vi "Load Program.vi"(7 "Queue in":refnum<queue>, 8 "error in (no error)":errorcluster, 9 "Program Filepath":path, 10 "HW Settings in":T7={"Bike Parameters"={"Bike Simulated?"=enum."Simulated", "COM Port"="", "Baud Rate"=0}, "Crank Motor Parameters"={"Crank Motor Simulated?"=enum."Simulated", "Crank Motor COM Port"="", "Unit ID"=0, "Baud Rate"=0, "Parity (Odd)"=enum."None", "Serial Type"=enum."RTU", "Flow Control (none)"=enum."None"}, "Resistance Parameters"={"Resistance Simulated?"=enum."Simulated", "Resistance COM Port"="", "Baud Rate"=0, "Flow Control (none)"=0, "Default Velocity (RPM)"=0.0, "Motor Address"=0, "Data Bits (8)"=0, "Parity (0:none)"=0, "Stop Bits"=0, "Resistance Motor Parameters"={"Command Mode"=0, "#Step/per Rev"=0, "Protocol Mode"=0, "Max Accel.(rev/sec/sec)"=0, "Jog Speed(rev/sec)"=0.0, "Decel Rate(rev/sec/sec)"=0, "Power Up Current(A)"=0.0, "Idle Current(A)"=0.0, "Position Fault(%)"=0, "Power Mode"=0, "Proportional Gain"=0.03, "Min Speed (rps)"=0.03, "Resistance Acceptance"=[]}, "Default Timeout (ms)"=0, "Log Resistance Motion"=FALSE}, "Acquisition Parameters"={"Acquisition Simulated?"=enum."Simulated", "Sample Rate"=0.0, "Torque AI Channel"="cDAQ1Mod1/ai0", "TC 1 Channel"="cDAQ1Mod2/ai0", "TC 2 Channel"="cDAQ1Mod2/ai0", "Torque CCW Polynomial Coeff (V to Nm)"=[], "Torque CW Polynomial Coeff (V to Nm)"=[], "Max Torque (Nm)"=0.0, "Min Torque (Nm)"=0.0, "B Input Terminal"="/cDAQ1Mod2/PFI1", "A Input Terminal"="/cDAQ1Mod2/PFI0", "Motor RPM Counter"="cDAQ1Mod2/ai0", "Motor Timing Counter"="cDAQ1Mod2/ctr0", "Motor Internal Output"="/cDAQ1/Ctr1InternalOutput", "Servo Encoder Pulses per Revolution"=2500, "Dyno Power Smoothing Time (s) for display only"=0.0, "Dyno Torque Tare Smoothing Time (s)"=2.0, "Power Error Smoothing Time (s) for display only"=0.0}, "Default Program Folder"=path "", "Program Filepath"=path "", "Program Changed?"=FALSE, "Plot Categories"=[]} {"Acquisition Parameters"."Power Error Smoothing Time (s) for display only" min=0.1; "Acquisition Parameters"."Dyno Power Smoothing Time (s) for display only" min=0.1; "Acquisition Parameters"."Torque CW Polynomial Coeff (V to Nm)" format="%.6e"; "Acquisition Parameters"."Torque CCW Polynomial Coeff (V to Nm)" format="%.6e"; "Resistance Parameters"."Stop Bits" items=["1.0"=10, "1.5"=15, "2.0"=20]; "Resistance Parameters"."Parity (0:none)" items=["None", "Odd", "Even", "Mark", "Space"]; "Resistance Parameters"."Data Bits (8)" min=5 max=8 step=1; "Resistance Parameters"."Flow Control (none)" items=["None", "XON/XOFF", "RTS/CTS", "XON/XOFF & RTS/CTS", "DTR/DSR", "XON/XOFF & DTR/DSR"]}, 11 "Program in":T1={"Raw Logging Configuration"={"Log File Base Path"=path ""}, "Sequence"={"Start RPM"=0.0, "End RPM"=0.0, "# RPM Steps"=0, "Dwell (s)"=0.0, "Start L-value / Resist"=0, "End L-value/Resist"=0, "# L-value/Resist Steps"=0, "Steady State +/-RPM"=0.0, "Enable Steady State +/- RPM"=FALSE, "Steady State Window (s)"=0.0, "Enable Steady State Max Wait"=FALSE, "Max Settle Time (s)"=0.0, "Enable Temperature Rest"=FALSE, "Rest TC2 threshold (degF)"=2.0, "Enable Max Time Rest"=FALSE, "Max Rest Time (s)"=10.0, "Rest RPM"=2.0, "RPM Ramp (rpm/s)"=10.0, "Resistance Motor Mode"=enum."v1 Bike"}, "Summary  CSV Log Configuration"={"Report  CSV File Path"=path "", "Enable Report CSV File"=FALSE}, "CSV Log Info"={"Report Title"="", "Time Stamp"=timestamp(0 s since 1904-01-01), "Serial Number"="", "Initial Temperature"=0.0, "Comments"=""}, "Table"=[]} {"Sequence"."RPM Ramp (rpm/s)" min=0.0 format="%#_6f"; "Sequence"."Rest RPM" min=0.0 format="%.1f"; "Sequence"."Max Rest Time (s)" min=0.0 format="%.1f"; "Sequence"."Rest TC2 threshold (degF)" format="%.1f"; "Sequence"."Max Settle Time (s)" min=0.0 format="%.1f"; "Sequence"."Steady State Window (s)" min=0.0 format="%.1f"; "Sequence"."Steady State +/-RPM" min=0.0 format="%.1f"; "Sequence"."# L-value/Resist Steps" min=1; "Sequence"."End L-value/Resist" min=0 max=100; "Sequence"."Start L-value / Resist" min=0 max=100; "Sequence"."Dwell (s)" min=0.0 format="%#_6f"; "Sequence"."# RPM Steps" min=1; "Sequence"."End RPM" min=0.0 max=200.0 format="%#_6f"; "Sequence"."Start RPM" min=0.0 max=200.0 format="%#_6f"}) -> (0 "error out":errorcluster, 2 "HW Settings out":T7={"Bike Parameters"={"Bike Simulated?"=enum."Simulated", "COM Port"="", "Baud Rate"=0}, "Crank Motor Parameters"={"Crank Motor Simulated?"=enum."Simulated", "Crank Motor COM Port"="", "Unit ID"=0, "Baud Rate"=0, "Parity (Odd)"=enum."None", "Serial Type"=enum."RTU", "Flow Control (none)"=enum."None"}, "Resistance Parameters"={"Resistance Simulated?"=enum."Simulated", "Resistance COM Port"="", "Baud Rate"=0, "Flow Control (none)"=0, "Default Velocity (RPM)"=0.0, "Motor Address"=0, "Data Bits (8)"=0, "Parity (0:none)"=0, "Stop Bits"=0, "Resistance Motor Parameters"={"Command Mode"=0, "#Step/per Rev"=0, "Protocol Mode"=0, "Max Accel.(rev/sec/sec)"=0, "Jog Speed(rev/sec)"=0.0, "Decel Rate(rev/sec/sec)"=0, "Power Up Current(A)"=0.0, "Idle Current(A)"=0.0, "Position Fault(%)"=0, "Power Mode"=0, "Proportional Gain"=0.03, "Min Speed (rps)"=0.03, "Resistance Acceptance"=[]}, "Default Timeout (ms)"=0, "Log Resistance Motion"=FALSE}, "Acquisition Parameters"={"Acquisition Simulated?"=enum."Simulated", "Sample Rate"=0.0, "Torque AI Channel"="cDAQ1Mod1/ai0", "TC 1 Channel"="cDAQ1Mod2/ai0", "TC 2 Channel"="cDAQ1Mod2/ai0", "Torque CCW Polynomial Coeff (V to Nm)"=[], "Torque CW Polynomial Coeff (V to Nm)"=[], "Max Torque (Nm)"=0.0, "Min Torque (Nm)"=0.0, "B Input Terminal"="/cDAQ1Mod2/PFI1", "A Input Terminal"="/cDAQ1Mod2/PFI0", "Motor RPM Counter"="cDAQ1Mod2/ai0", "Motor Timing Counter"="cDAQ1Mod2/ctr0", "Motor Internal Output"="/cDAQ1/Ctr1InternalOutput", "Servo Encoder Pulses per Revolution"=2500, "Dyno Power Smoothing Time (s) for display only"=0.0, "Dyno Torque Tare Smoothing Time (s)"=2.0, "Power Error Smoothing Time (s) for display only"=0.0}, "Default Program Folder"=path "", "Program Filepath"=path "", "Program Changed?"=FALSE, "Plot Categories"=[]} {"Acquisition Parameters"."Power Error Smoothing Time (s) for display only" min=0.1; "Acquisition Parameters"."Dyno Power Smoothing Time (s) for display only" min=0.1; "Acquisition Parameters"."Torque CW Polynomial Coeff (V to Nm)" format="%.6e"; "Acquisition Parameters"."Torque CCW Polynomial Coeff (V to Nm)" format="%.6e"; "Resistance Parameters"."Stop Bits" items=["1.0"=10, "1.5"=15, "2.0"=20]; "Resistance Parameters"."Parity (0:none)" items=["None", "Odd", "Even", "Mark", "Space"]; "Resistance Parameters"."Data Bits (8)" min=5 max=8 step=1; "Resistance Parameters"."Flow Control (none)" items=["None", "XON/XOFF", "RTS/CTS", "XON/XOFF & RTS/CTS", "DTR/DSR", "XON/XOFF & DTR/DSR"]}, 3 "Program out":T1={"Raw Logging Configuration"={"Log File Base Path"=path ""}, "Sequence"={"Start RPM"=0.0, "End RPM"=0.0, "# RPM Steps"=0, "Dwell (s)"=0.0, "Start L-value / Resist"=0, "End L-value/Resist"=0, "# L-value/Resist Steps"=0, "Steady State +/-RPM"=0.0, "Enable Steady State +/- RPM"=FALSE, "Steady State Window (s)"=0.0, "Enable Steady State Max Wait"=FALSE, "Max Settle Time (s)"=0.0, "Enable Temperature Rest"=FALSE, "Rest TC2 threshold (degF)"=2.0, "Enable Max Time Rest"=FALSE, "Max Rest Time (s)"=10.0, "Rest RPM"=2.0, "RPM Ramp (rpm/s)"=10.0, "Resistance Motor Mode"=enum."v1 Bike"}, "Summary  CSV Log Configuration"={"Report  CSV File Path"=path "", "Enable Report CSV File"=FALSE}, "CSV Log Info"={"Report Title"="", "Time Stamp"=timestamp(0 s since 1904-01-01), "Serial Number"="", "Initial Temperature"=0.0, "Comments"=""}, "Table"=[]} {"Sequence"."RPM Ramp (rpm/s)" min=0.0 format="%#_6f"; "Sequence"."Rest RPM" min=0.0 format="%.1f"; "Sequence"."Max Rest Time (s)" min=0.0 format="%.1f"; "Sequence"."Rest TC2 threshold (degF)" format="%.1f"; "Sequence"."Max Settle Time (s)" min=0.0 format="%.1f"; "Sequence"."Steady State Window (s)" min=0.0 format="%.1f"; "Sequence"."Steady State +/-RPM" min=0.0 format="%.1f"; "Sequence"."# L-value/Resist Steps" min=1; "Sequence"."End L-value/Resist" min=0 max=100; "Sequence"."Start L-value / Resist" min=0 max=100; "Sequence"."Dwell (s)" min=0.0 format="%#_6f"; "Sequence"."# RPM Steps" min=1; "Sequence"."End RPM" min=0.0 max=200.0 format="%#_6f"; "Sequence"."Start RPM" min=0.0 max=200.0 format="%#_6f"})   [LabVIEW 2021, in "Config Module.lvlib"]
uses:
  Config Module.lvlib
  Controls/Config File Operation Enum.ctl
  support/Message Queue/Enqueue Message (Single).vi
  support/Message Queue/Message Cluster.ctl
  Peloton Bike/Signal Type.ctl
  Peloton Bike/Bike Parameters.ctl
  Crank Motor/Signal Type.ctl
  Crank Motor/Crank Motor Parameters.ctl
  Resistance Motor/Signal Type.ctl
  Resistance Motor/Resistance Motor Default Params.ctl
  Resistance Motor/Resistance Parameters.ctl
  Acquisition/Signal Type.ctl
  Acquisition/Acquisition Parameters.ctl
  Settings/Settings.ctl
  Settings/Settings.lvlib
  Logging/Logging Configuration.ctl
  Logging/Logging.lvlib
  Settings/Sequence Cluster.ctl
  controls/CSV Log Cluster.ctl
  Settings/Program Cluster.ctl
  controls/CSV Log Info Cluster.ctl
  Graph Folder/History Graph/Controls/Plot Category Cluster.ctl
  Resistance Motor/Resistance Mode Enum.ctl
  Resistance Motor/Resistance Acceptance Range.ctl
panel:
  # "Settled when"
  # "RPM is within"
  # "RPM of set RPM for last"
  # "seconds"
  # "OR"
  # "seconds since last step change"
  # "More than"
  # "Rest at end of each step at"
  # "RPM until"
  # "TC2 temperature is below"
  # "deg F"
  # "OR"
  # "seconds have elapsed"
  # "More than"
  # "Settled when"
  # "RPM is within"
  # "RPM of set RPM for last"
  # "seconds"
  # "OR"
  # "seconds since last step change"
  # "More than"
  # "Rest at end of each step at"
  # "RPM until"
  # "TC2 temperature is below"
  # "deg F"
  # "OR"
  # "seconds have elapsed"
  # "More than"
  # "(Silicon Labs CP210x)"
  # "(Silicon Labs CP210x)"
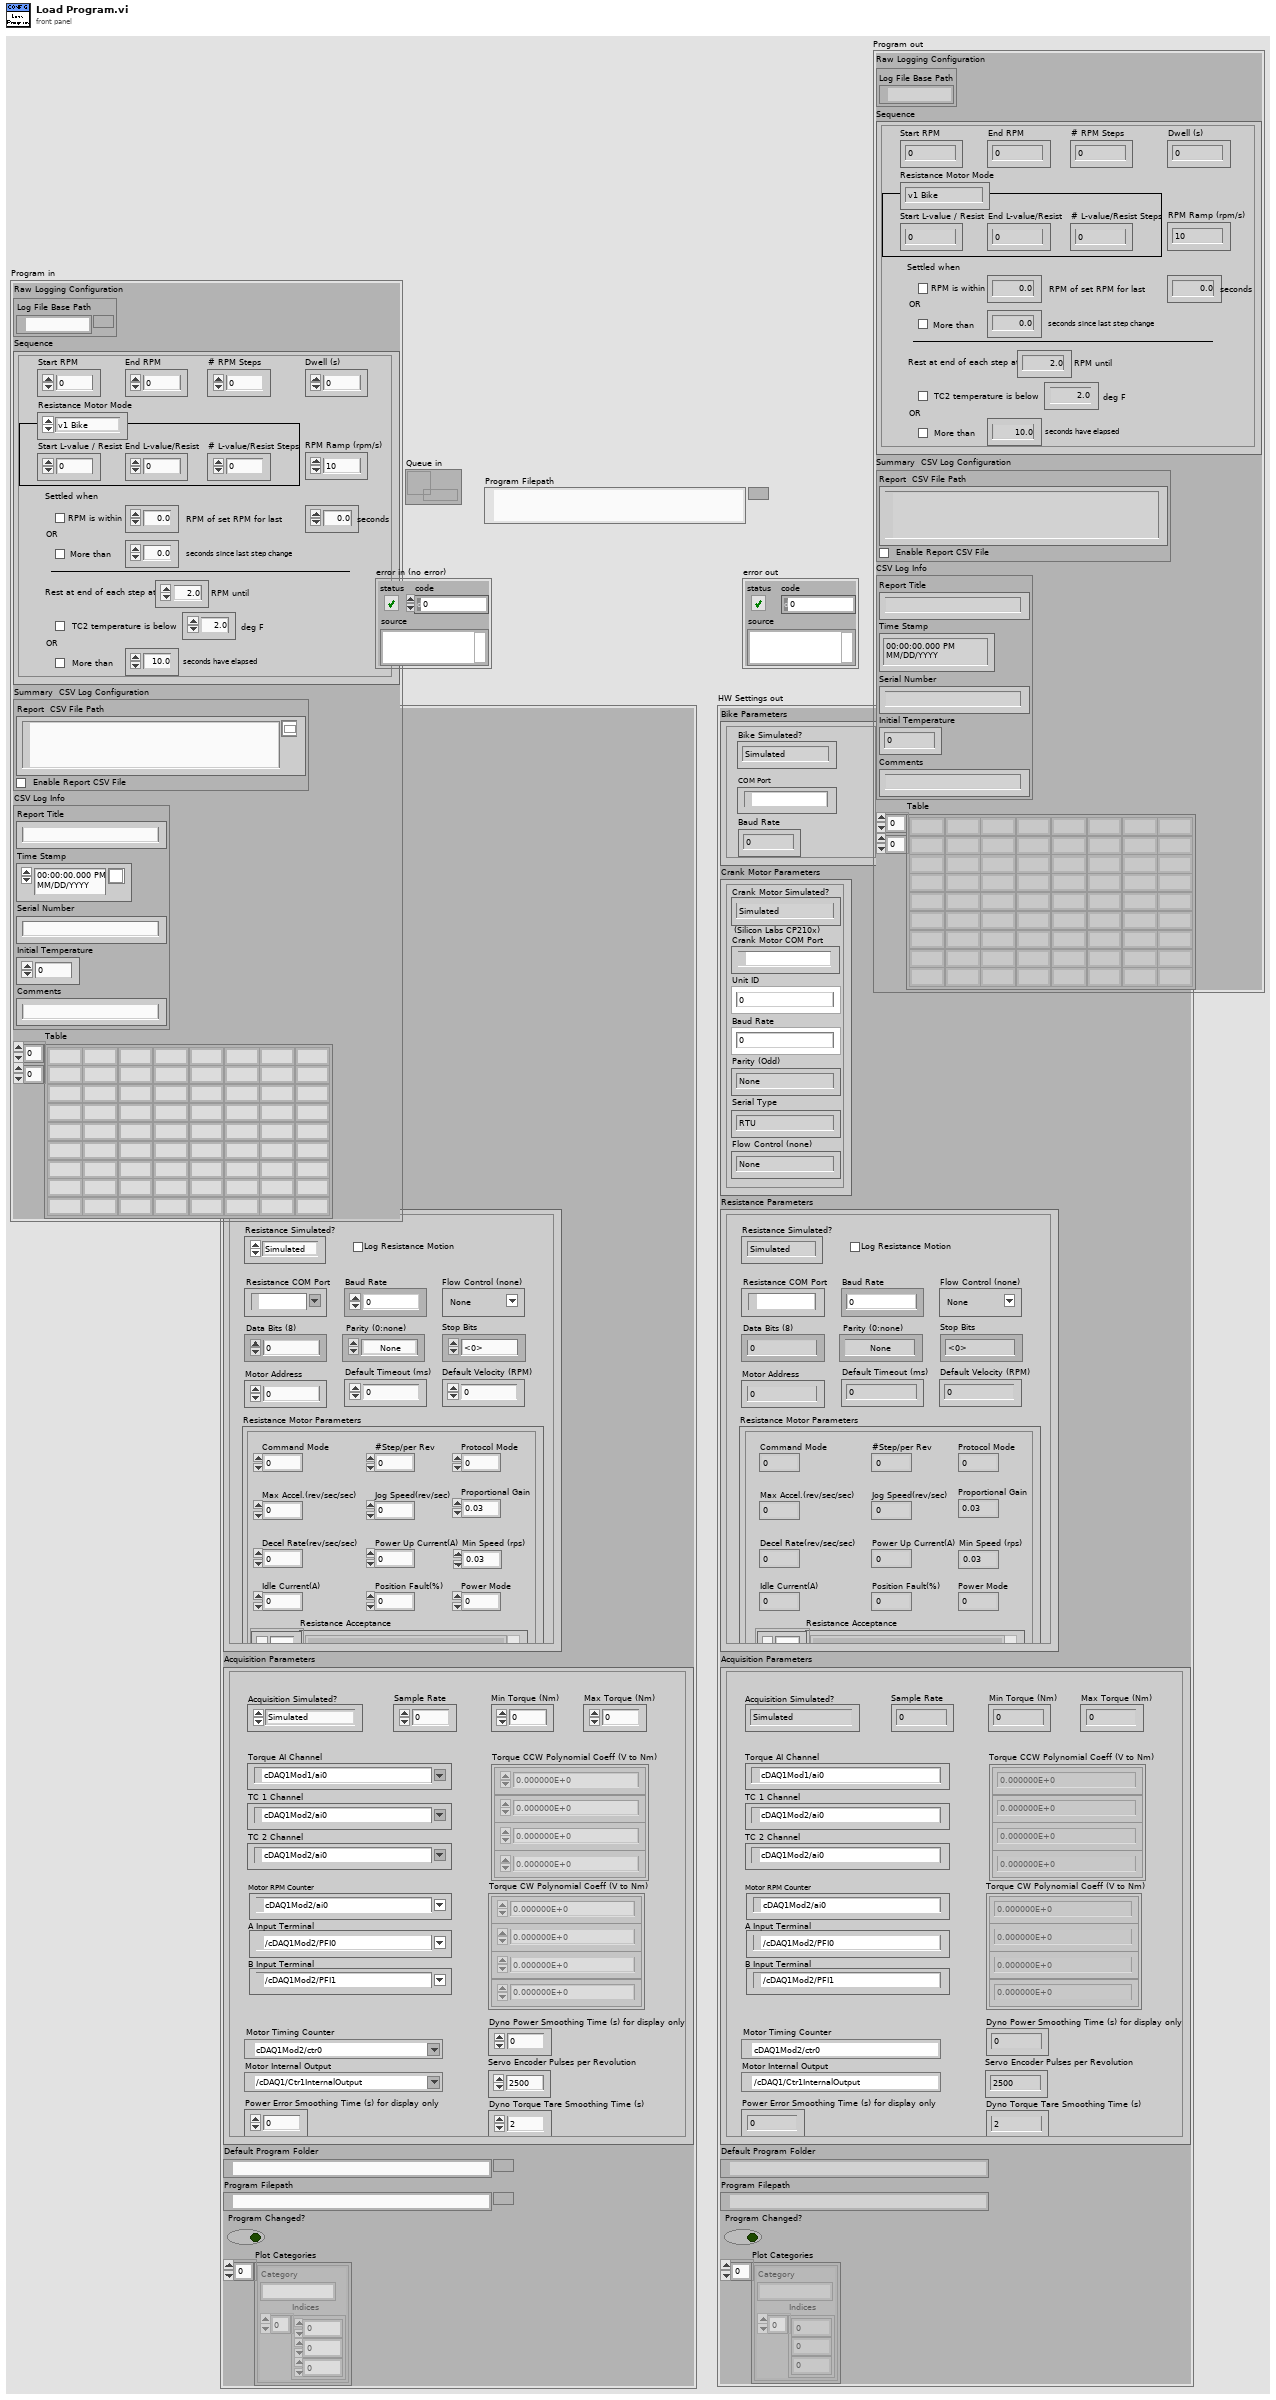
[diagram p1: front panel]
types:
  T1 = typedef "Settings.lvlib/Program Cluster.ctl" = cluster{"Raw Logging Configuration":T2, "Sequence":T3, "Summary  CSV Log Configuration":T5, "CSV Log Info":T6, "Table":string[][]}
  T2 = typedef "Logging.lvlib/Logging Configuration.ctl" = cluster{"Log File Base Path":path}
  T3 = typedef "Sequence Cluster.ctl" = cluster{"Start RPM":dbl, "End RPM":dbl, "# RPM Steps":i32, "Dwell (s)":dbl, "Start L-value / Resist":i32, "End L-value/Resist":i32, "# L-value/Resist Steps":i32, "Steady State +/-RPM":dbl, "Enable Steady State +/- RPM":bool, "Steady State Window (s)":dbl, "Enable Steady State Max Wait":bool, "Max Settle Time (s)":dbl, "Enable Temperature Rest":bool, "Rest TC2 threshold (degF)":dbl, "Enable Max Time Rest":bool, "Max Rest Time (s)":dbl, "Rest RPM":dbl, "RPM Ramp (rpm/s)":dbl, "Resistance Motor Mode":T4}
  T4 = typedef "Resistance Mode Enum.ctl" = enum16{"v1 Bike", "v1.5 Bike", "Disabled"}
  T5 = typedef "CSV Log Cluster.ctl" = cluster{"Report  CSV File Path":path, "Enable Report CSV File":bool}
  T6 = typedef "CSV Log Info Cluster.ctl" = cluster{"Report Title":string, "Time Stamp":timestamp, "Serial Number":string, "Initial Temperature":dbl, "Comments":string}
  T7 = typedef "Settings.lvlib/Settings.ctl" = cluster{"Bike Parameters":T8, "Crank Motor Parameters":T10, "Resistance Parameters":T12, "Acquisition Parameters":T16, "Default Program Folder":path, "Program Filepath":path, "Program Changed?":bool, "Plot Categories":T18[]}
  T8 = typedef "Bike Parameters.ctl" = cluster{"Bike Simulated?":T9, "COM Port":refnum<visa-resource-name>, "Baud Rate":u32}
  T9 = typedef "Peloton Bike.lvlib/Signal Type.ctl" = enum16{"Simulated", "Real"}
  T10 = typedef "Crank Motor Parameters.ctl" = cluster{"Crank Motor Simulated?":T11, "Crank Motor COM Port":refnum<visa-resource-name>, "Unit ID":u8, "Baud Rate":u32, "Parity (Odd)":enum16{"None", "Odd", "Even", "Mark", "Space"}, "Serial Type":enum16{"RTU", "ASCII"}, "Flow Control (none)":enum16{"None", "XON/XOFF", "RTS/CTS", "XON/XOFF & RTS/CTS", "DTR/DSR", "XON/XOFF & DTR/DSR"}}
  T11 = typedef "Crank Motor.lvlib/Signal Type.ctl" = enum16{"Simulated", "Real"}
  T12 = typedef "Resistance Parameters.ctl" = cluster{"Resistance Simulated?":T13, "Resistance COM Port":refnum<visa-resource-name>, "Baud Rate":u32, "Flow Control (none)":u16, "Default Velocity (RPM)":dbl, "Motor Address":i32, "Data Bits (8)":u16, "Parity (0:none)":u16, "Stop Bits":u16, "Resistance Motor Parameters":T14, "Default Timeout (ms)":i32, "Log Resistance Motion":bool}
  T13 = typedef "Resistance Motor.lvlib/Signal Type.ctl" = enum16{"Simulated", "Real"}
  T14 = typedef "Resistance Motor.lvlib/Resistance Motor Default Params.ctl" = cluster{"Command Mode":u16, "#Step/per Rev":u16, "Protocol Mode":u16, "Max Accel.(rev/sec/sec)":u16, "Jog Speed(rev/sec)":dbl, "Decel Rate(rev/sec/sec)":u16, "Power Up Current(A)":dbl, "Idle Current(A)":dbl, "Position Fault(%)":u16, "Power Mode":u16, "Proportional Gain":dbl, "Min Speed (rps)":dbl, "Resistance Acceptance":T15[]}
  T15 = typedef "Resistance Acceptance Range.ctl" = cluster{"Range Min.":i32, "Range Max.":i32, "+/- Tolerance":i32}
  T16 = typedef "Acquisition.lvlib/Acquisition Parameters.ctl" = cluster{"Acquisition Simulated?":T17, "Sample Rate":dbl, "Torque AI Channel":tag, "TC 1 Channel":tag, "TC 2 Channel":tag, "Torque CCW Polynomial Coeff (V to Nm)":dbl[], "Torque CW Polynomial Coeff (V to Nm)":dbl[], "Max Torque (Nm)":dbl, "Min Torque (Nm)":dbl, "B Input Terminal":tag, "A Input Terminal":tag, "Motor RPM Counter":tag, "Motor Timing Counter":tag, "Motor Internal Output":tag, "Servo Encoder Pulses per Revolution":u32, "Dyno Power Smoothing Time (s) for display only":dbl, "Dyno Torque Tare Smoothing Time (s)":dbl, "Power Error Smoothing Time (s) for display only":dbl}
  T17 = typedef "Acquisition.lvlib/Signal Type.ctl" = enum16{"Simulated", "Real"}
  T18 = typedef "History Graph.lvclass/Plot Category Cluster.ctl" = cluster{"Category":string, "Indices":i32[]}
  T19 = typedef "Config Module.lvlib/Config File Operation Enum.ctl" = enum16{"Read", "Write"}
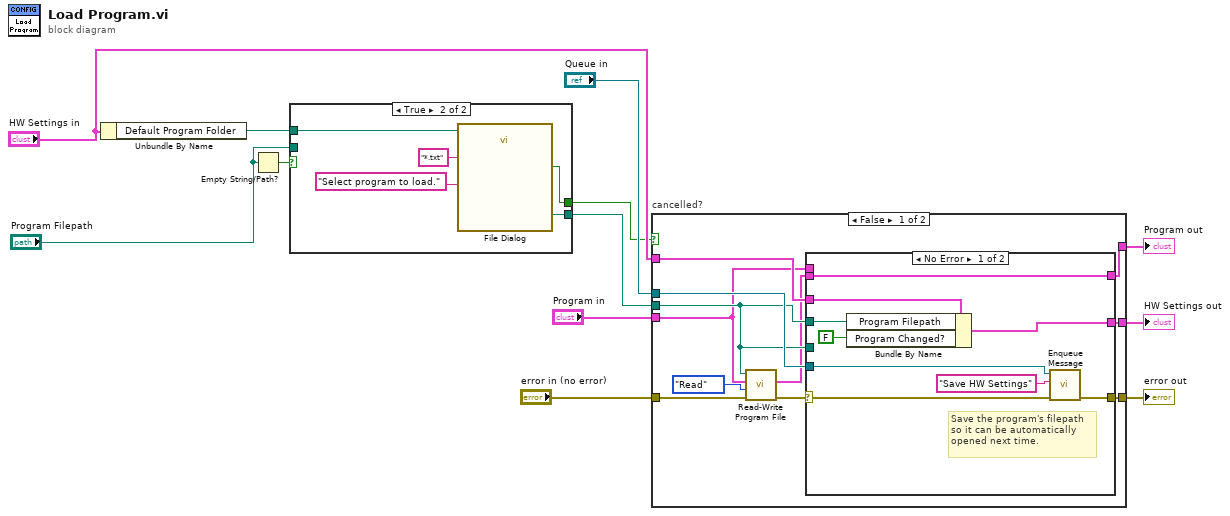
[diagram p0: block diagram]
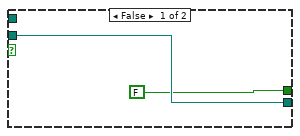
[diagram p2: hidden frame]
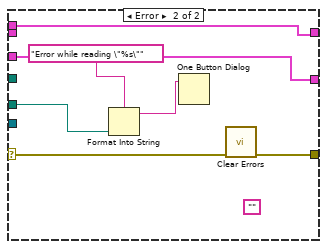
[diagram p3: hidden frame]
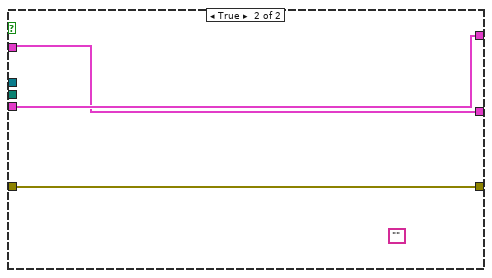
[diagram p4: hidden frame]
diagram:
  n1 = Unbundle By Name("HW Settings in") -> ("Default Program Folder"=w4:path)
  n2 = Empty String/Path?(string/path="Program Filepath") -> (empty?=w3:bool)
  n3 = case shown="True" w3 {
    tunnel: w4 -> [_ w19]
    tunnel: [FALSE ("cancelled") w18] -> w6
    tunnel: [w14 w17] -> w9
    tunnel: "Program Filepath" -> [w14 _]
    frame False {
    }
    frame True {
      n4 = call "File Dialog"("start path"=w19, "prompt"="Select program to load.", "pattern (all files)"="*.txt") -> ("selected path"=w17:path, "cancelled"=w18:bool)  [unwired: 9 in, 2 out]
    }
  }
  n5 = case "cancelled?" shown="False" w6 {
    tunnel: "error in (no error)" -> [w30 w49]
    tunnel: [w25 w49] -> w2
    tunnel: "Program in" -> [w20 w48]
    tunnel: [w21 w48] -> w8
    tunnel: w9 -> [w23 _]
    tunnel: "HW Settings in" -> [w28 w47]
    tunnel: [w27 w47] -> w11
    tunnel: "Queue in" -> [w24 _]
    frame False {
      n6 = call "Read-Write Program File.vi"("configuration file path"=w23, "Program in"=w20, "Mode"=Config_File_Operation_Enum."Read", "error in"=w30) -> ("Program out"=w22:T1, "error out"=w26:errorcluster)  [unwired: 4 in, 1 out]
      n7 = case shown="No Error" w26 {
        selector: w26 -> [w36 w42]
        tunnel: w28 -> [w39 w46]
        tunnel: [w38 w46] -> w27
        tunnel: w23 -> [w33 _]
        tunnel: [w35 w41] -> w25
        tunnel: w24 -> [w34 _]
        tunnel: w23 -> [_ w44]
        tunnel: [w31 w40] -> w21
        tunnel: w22 -> [w31 _]
        tunnel: w20 -> [_ w40]
        frame No Error {
          # "Save the program's filepath\nso it can be automatically\nopened next time."
          n8 = Bundle By Name(cluster=w39, "Program Filepath"=w33, "Program Changed?"=FALSE) -> (w38:T7)
          n9 = call-poly "Enqueue Message.vi"("error in (no error)"=w36, "Message"="Save HW Settings", "Message Queue"=w34) -> ("error out"=w35:errorcluster)  [unwired: 7 in, 1 out]
        }
        frame Error {
          (unwired) ""
          n10 = Format Into String(format string="Error while reading \"%s\"", w44) -> (resulting string=w43:string)  [unwired: 2 in, 1 out]
          n11 = One Button Dialog(message=w43) -> ()  [unwired: 1 in, 1 out]
          n12 = call <vilib>:"Clear Errors.vi"("error in (no error)"=w42) -> ("error out"=w41:errorcluster)  [unwired: 5 in, 1 out]
        }
      }
    }
    frame True {
      (unwired) ""
    }
  }
  "HW Settings out" <- w11
  "Program out" <- w8
  "error out" <- w2
